vi "Package Data.vi"(8 "error in":errorcluster, 10 "DataIn":string, 11 "P in":refnum<class "P.lvclass">) -> (0 "error out":errorcluster, 3 "P out":refnum<class "P.lvclass">)   [LabVIEW 2015, in "P.lvclass"]
uses:
  P.lvclass
  P.lvclass/P.ctl
  Write P.vi
  Reusable/Data/Write measTime.vi
  <vilib>/gmath/NI_Gmath.lvlib
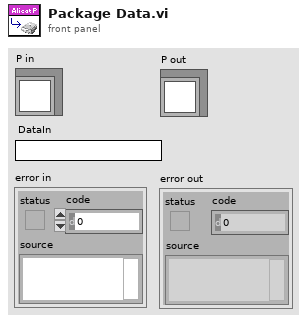
[diagram p1: front panel]
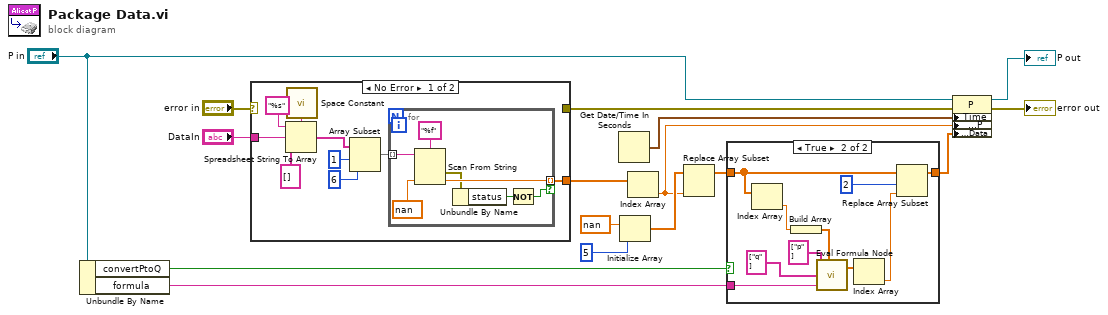
[diagram p0: block diagram]
diagram:
  n1 = Unbundle By Name("P in") -> ("convertPtoQ"=w4:bool, "formula"=w3:string)
  n2 = case shown="No Error" "error in" {
    selector: "error in" -> [_ w33]
    tunnel: "DataIn" -> [w22 _]
    tunnel: [w18 _] -> w10
    tunnel: [_ w33] -> w7
    frame No Error {
      n3 = call <vilib>:"Space Constant.vi"() -> ("String"=w24:string)
      n4 = Spreadsheet String To Array(delimiter (Tab)=w24, format string="%s", spreadsheet string=w22, array type (2D Dbl)=string[] []) -> (array=w21:string[])
      n5 = Array Subset(array=w21, index=1, length=6) -> (w19:string[])
      n6 = for {
        tunnel: w19 -> [w29] mode=indexing
        tunnel: [w30] -> w18 mode=indexing if=w26
        n7 = Scan From String(format string="%f", input string=w29, default 1=sgl nan ("default value 1")) -> (error out=w28:errorcluster, output 1=w30:sgl)  [unwired: 2 in, 2 out]
        n8 = Unbundle By Name(w28) -> ("status"=w27:bool)
        n9 = Not(x=w27) -> (.not. x?=w26:bool)
      }
    }
    frame Error {
    }
  }
  n10 = Get Date/Time In Seconds() -> (seconds since 1Jan1904=w14:timestamp)
  n11 = Initialize Array(nan ("element"), 5 ("dimension size")) -> (w9:dbl[])
  n12 = Index Array(array=w10) -> (element=w6:sgl)  [unwired: 1 in]
  n13 = Replace Array Subset(array=w9, new element=w6) -> (w2:dbl[])  [unwired: 1 in]
  n14 = case shown="True" w4 {
    tunnel: w3 -> [_ w42]
    tunnel: w2 -> [w34 w37]
    tunnel: [w34 w35] -> w1
    frame False {
    }
    frame True {
      n15 = Index Array(array=w37) -> (element=w41:dbl)  [unwired: 1 in]
      n16 = Build Array(w41) -> (w40:dbl[])
      n17 = call <vilib>:"Eval Formula Node.vi"("Variables Input"=string[] ["p"] ("Variables Output"), "Input Values"=w40, "Variables Output"=string[] ["q"], "formula"=w42) -> ("Output Values"=w39:dbl[])  [unwired: 1 in, 1 out]
      n18 = Index Array(array=w39) -> (element=w38:dbl)  [unwired: 1 in]
      n19 = Replace Array Subset(array=w37, new element=w38, index=2) -> (w35:dbl[])
    }
  }
  n20 = property class="P"(reference="P in", error in=w7, "Time"=w14, "Accessors:P"=w6, "Accessors:Data"=w1) -> (reference out=→"P out":refnum<class "P.lvclass">, error out=→"error out":errorcluster)
